vi "Initialise.vi"(8 "error in (no error)":errorcluster) -> (0 "error out":errorcluster, 3 "Clock Generator":refnum<class "Clock Generator.lvclass">)   [LabVIEW 2021, in "Clock Generator.lvclass"]
uses:
  Clock Generator.lvclass
  Clock Generator.lvclass/Clock Generator.ctl
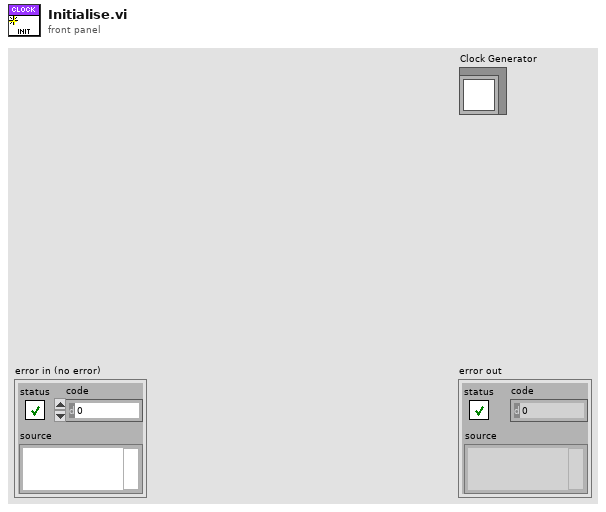
[diagram p1: front panel]
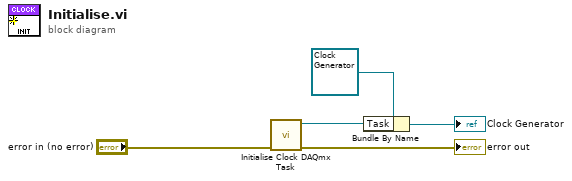
[diagram p0: block diagram]
diagram:
  n1 = call "Initialise Clock DAQmx Task.vi"("error in"="error in (no error)") -> ("error out"=→"error out":errorcluster, "task out"=w5:refnum<k21>)  [unwired: 9 in]
  n2 = Bundle By Name(cluster=refnum<class "Clock Generator.lvclass"> refnum ("Clock Generator out"), "Task"=w5) -> (→"Clock Generator":refnum<class "Clock Generator.lvclass">)
